vi "MagBoard_n128_Serial_FileIO.vi"(5 "Serial Settings":T1={"baud rate"=115200, "data bits"=8, "parity"=enum."None", "stop bits"=10, "flow control"=0} {"flow control" items=["None"=0, "XON/XOFF"=1, "RTS/CTS"=2, "DTR/DSR"=4]; "stop bits" items=["1.0"=10, "1.5"=15, "2.0"=20]; "data bits" min=5 max=8 step=1; "baud rate" items=["75"=75, "110"=110, "134"=134, "150"=150, "300"=300, "600"=600, "1200"=1200, "1800"=1800, "2400"=2400, "4800"=4800, "7200"=7200, "9600"=9600, "14400"=14400, "19200"=19200, "28800"=28800, "38400"=38400, "56000"=56000, "57600"=57600, "115200"=115200, "128000"=128000, "230400"=230400]}, 7 "VISA resource name":refnum<visa-resource-name>="COM16", 9 "File_Code":string, 10 "Directory":path, 11 "Remote Filename":string) -> (0 "error out":errorcluster, 2 "FilePath Out":path, 3 "Packets Recieved":i32)   [LabVIEW 2018]
panel:
  in  "Tab Control":enum32{"Display", "Debug", "Configuration"}(tab)
  out "Save Progress":i16(slide) scale=0.0..975.0
  out "Reading":bool
  out "Input Data":string
  out "read count":u32
  out "offset byte?":string
  out "Connected":bool
  out "EOF?":bool
  out "Initialised":bool
  # "scapes: Saving..."
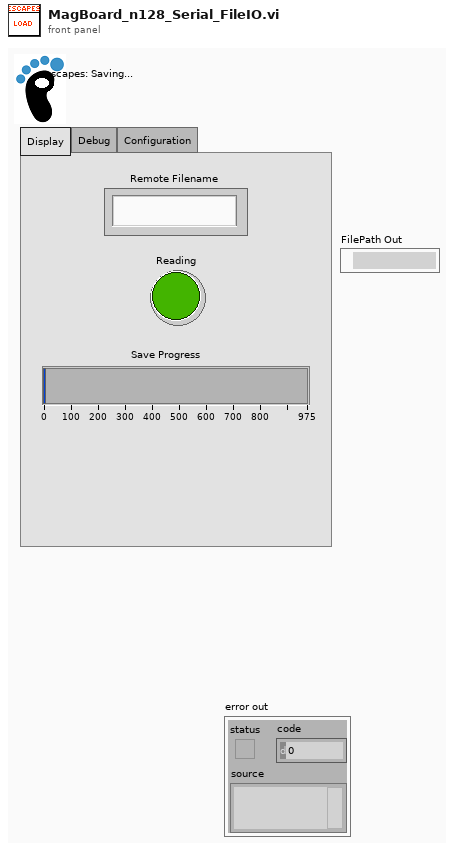
[diagram p1: front panel]
types:
  T1 = cluster{"baud rate":u32, "data bits":u16, "parity":enum16{"None", "Odd", "Even", "Mark", "Space"}, "stop bits":u16, "flow control":u16}
  T2 = enum16{"open", "replace", "create", "open or create", "replace or create", "replace or create with confirmation"}
  T3 = enum16{"big-endian, network order", "native, host order", "little-endian"}
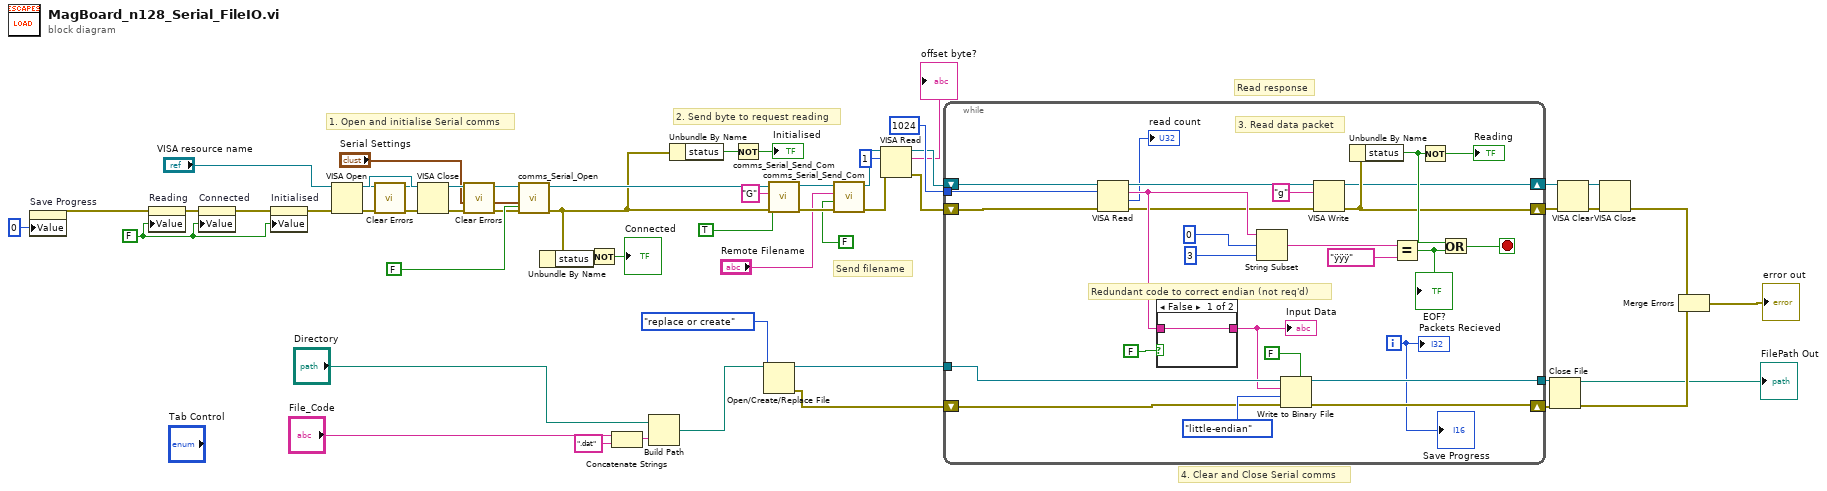
[diagram p0: block diagram]
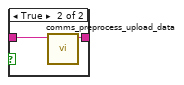
[diagram p2: hidden frame]
diagram:
  w40 = FALSE ("Send Init Comm?")
  # "Send filename"
  # "2. Send byte to request reading"
  # "Read response"
  # "4. Clear and Close Serial comms"
  # "1. Open and initialise Serial comms"
  n1 = property on="Save Progress" class="Slide (strict)"("Value"=i16 0 ("Save Progress")) -> (error out=w2:errorcluster)  [unwired: 2 in, 1 out]
  n2 = property on="Reading" class="Bool (strict)"(error in=w2, "Value"=w40) -> (error out=w41:errorcluster)  [unwired: 1 in, 1 out]
  n3 = property on="Connected" class="Bool (strict)"(error in=w41, "Value"=w40) -> (error out=w42:errorcluster)  [unwired: 1 in, 1 out]
  n4 = property on="Initialised" class="Bool (strict)"(error in=w42, "Value"=w40) -> (error out=w30:errorcluster)  [unwired: 1 in, 1 out]
  n5 = VISA Open(error in (no error)=w30, VISA resource name="VISA resource name") -> (VISA resource name=w39:refnum<visa-resource-name>, error out=w38:errorcluster)  [unwired: 3 in]
  n6 = call <vilib>:"Clear Errors.vi"("error in (no error)"=w38) -> ("error out"=w37:errorcluster)  [unwired: 5 in, 1 out]
  n7 = VISA Close(VISA resource name=w39, error in (no error)=w37) -> (error out=w36:errorcluster)
  n8 = call <vilib>:"Clear Errors.vi"("error in (no error)"=w36) -> ("error out"=w35:errorcluster)  [unwired: 5 in, 1 out]
  n9 = call "comms_Serial_Open.vi"("Send Init Comm?"=FALSE, "error in (no error)"=w35, "Serial Settings in"="Serial Settings", "VISA Refnum in"="VISA resource name") -> ("error out"=w24:errorcluster, "VISA Refnum out"=w25:refnum<visa-resource-name>)  [unwired: 5 in, 1 out]
  n10 = Unbundle By Name(w24) -> ("status"=w46:bool)
  n11 = Not(x=w46) -> (.not. x?=→"Connected":bool)
  n12 = Concatenate Strings("File_Code", ".dat" ("string")) -> (w8:string)
  n13 = Build Path(base path="Directory", name or relative path=w8) -> (appended path=w4:path)
  n14 = Unbundle By Name(w24) -> ("status"=w45:bool)
  n15 = Not(x=w45) -> (.not. x?=→"Initialised":bool)
  n16 = Open/Create/Replace File(file path (use dialog)=w4, operation (0:open)=T2."replace or create") -> (refnum out=w22:refnum<file>, error out=w21:errorcluster)  [unwired: 4 in, 1 out]
  n17 = call "comms_Serial_Send_Com.vi"("error in"=w24, "Buffer Clear?"=TRUE, "Command"="G", "VISA resource in"=w25) -> ("error out"=w29:errorcluster, "VISA resource Out"=w27:refnum<visa-resource-name>)  [unwired: 5 in, 1 out]
  n18 = call "comms_Serial_Send_Com.vi"("error in"=w29, "Buffer Clear?"=FALSE, "Command"="Remote Filename", "VISA resource in"=w27) -> ("error out"=w10:errorcluster, "VISA resource Out"=w17:refnum<visa-resource-name>)  [unwired: 5 in, 1 out]
  n19 = VISA Read(VISA resource name=w17, byte count=u32 1, error in (no error)=w10) -> (VISA resource name out=w16:refnum<visa-resource-name>, read buffer=→"offset byte?":string, error out=w11:errorcluster)  [unwired: 1 out]
  n20 = while {
    shift-right: [w68] -> w48
    shift-left: w16 -> [w66]
    shift-right: [w70] -> w47
    shift-left: w11 -> [w65]
    tunnel: u32 1024 ("byte count") -> [w73]
    tunnel: w22 -> [w63]
    shift-right: [w62] -> w20
    shift-left: w21 -> [w55]
    tunnel: [w60] -> w19
    i -> [w52]
    stop <- w75 stop-if-true
    # "Redundant code to correct endian (not req'd)"
    # "3. Read data packet"
    n21 = VISA Read(VISA resource name=w66, byte count=w73, error in (no error)=w65) -> (VISA resource name out=w69:refnum<visa-resource-name>, read buffer=w58:string, return count=→"read count":u32, error out=w54:errorcluster)
    n22 = case shown="False" FALSE {
      tunnel: w58 -> [w79 w81]
      tunnel: [w79 w80] -> w57
      frame False {
      }
      frame True {
        n23 = call "comms_preprocess_upload_data.vi"("Binary Input Data"=w81) -> ("Binary Output (string)"=w80:string)  [unwired: 10 in]
      }
    }
    "Input Data" <- w57
    n24 = String Subset(string=w58, offset (0)=0, length (rest)=3 ("length (rest)")) -> (substring=w71:string)
    n25 = Write to Binary File(file (use dialog)=w63, data=w57, error in=w55, 5:FALSE ("prepend array or string size? (T)"), 9:T3."little-endian" ("byte order (0:big-endian, network order)")) -> (refnum out=w60:refnum<file>, error out=w62:errorcluster)  [unwired: 1 in, 1 out]
    n26 = VISA Write(VISA resource name=w69, write buffer="g", error in (no error)=w54) -> (VISA resource name out=w68:refnum<visa-resource-name>, error out=w70:errorcluster)  [unwired: 1 out]
    n27 = Unbundle By Name(w70) -> ("status"=w74:bool)
    n28 = Equal?(x=w71, y="ÿÿÿ") -> (x = y?=w76:bool)
    "EOF?" <- w76
    n29 = Not(x=w74) -> (.not. x?=→"Reading":bool)
    n30 = Or(x=w74, y=w76) -> (x .or. y?=w75:bool)
    "Packets Recieved" <- w52
    "Save Progress" <- w52
  }
  n31 = Close File(refnum=w19, error in=w20) -> (path=→"FilePath Out":path, error out=w12:errorcluster)
  n32 = VISA Clear(VISA resource name=w48, error in (no error)=w47) -> (VISA resource name out=w50:refnum<visa-resource-name>, error out=w49:errorcluster)
  n33 = VISA Close(VISA resource name=w50, error in (no error)=w49) -> (error out=w13:errorcluster)
  n34 = Merge Errors(w13, w12) -> (→"error out":errorcluster)
